vi "SetImageFromLVImageData_Greyscale.vi"(10 "LV Image Data":T1, 11 "Greyscale Image":refnum<data-value>) -> (3 "Greyscale Image (duplicate)":refnum<data-value>)   [LabVIEW 2020, in "g_ar_toolkit.lvlib"]
uses:
  g_ar_toolkit.lvlib
  <vilib>/picture/picture.llb/imagedata.ctl
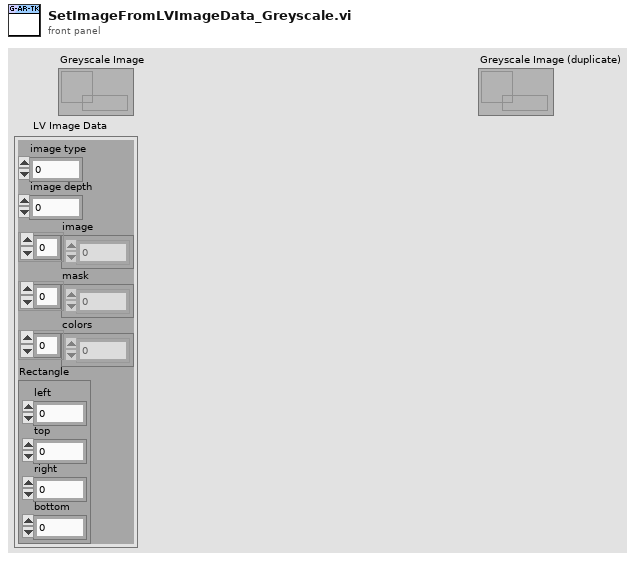
[diagram p1: front panel]
types:
  T1 = typedef "imagedata.ctl" = cluster{"image type":i32, "image depth":i32, "image":u8[], "mask":u8[], "colors":u32[], "Rectangle":cluster{"left":i16, "top":i16, "right":i16, "bottom":i16}}
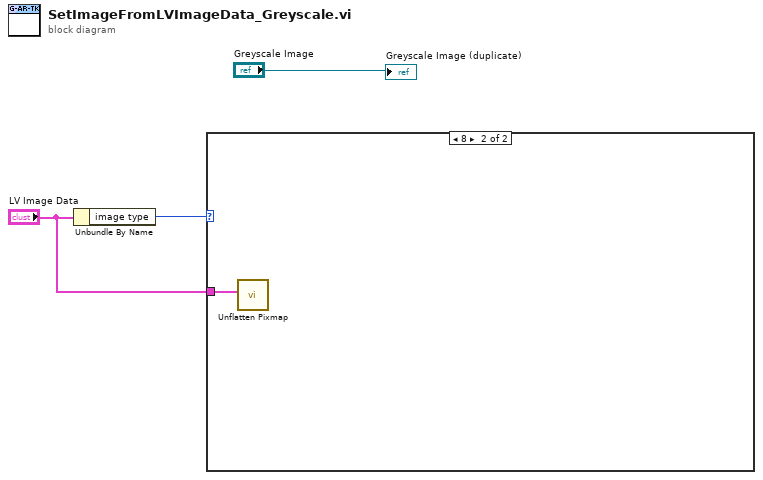
[diagram p0: block diagram]
diagram:
  n1 = Unbundle By Name("LV Image Data") -> ("image type"=w2:i32)
  n2 = case shown="8" w2 {
    tunnel: "LV Image Data" -> [_ w4]
    frame 0, Default {
    }
    frame 8 {
      n3 = call <vilib>:"Unflatten Pixmap.vi"("image data"=w4) -> ()  [unwired: 4 in, 7 out]
    }
  }
  "Greyscale Image (duplicate)" <- "Greyscale Image"
